vi "LTVUnicycleCtrl_New.vi"(8 "Max Velocity":dbl=9.0, 9 "dT":dbl=0.02, 10 "RELMS":T6=[[1.0], [2.0]], 11 "QELMS":T6=[[0.0625], [0.125], [0.2]]) -> (0 "Error":bool, 3 "LTV_UNICYCLE_CONTROLLER":T1={"States"=0, "Inputs"=0, "PoseError"={"TRANSLATION"={"X"=0.0, "Y"=0.0}, "ROTATION"={"VALUE"=0.0, "COS"=1.0, "SIN"=0.0}}, "PoseTolerance"={"TRANSLATION"={"X"=0.0, "Y"=0.0}, "ROTATION"={"VALUE"=0.0, "COS"=1.0, "SIN"=0.0}}, "Dt"=0.02, "Enabled"=FALSE, "LQR_K_Table"={"Table Xs"=[], "Table Ys"=[], "MinX"=0.0, "MaxX"=0.0, "ItemCount"=0, "Rows"=0, "Columns"=0}} {"PoseTolerance"."ROTATION"."SIN" format="%13.4f"; "PoseTolerance"."ROTATION"."COS" format="%13.4f"; "PoseTolerance"."ROTATION"."VALUE" format="%13.4f"; "PoseTolerance"."TRANSLATION"."Y" format="%14.3f"; "PoseTolerance"."TRANSLATION"."X" format="%14.3f"; "PoseError"."ROTATION"."SIN" format="%13.4f"; "PoseError"."ROTATION"."COS" format="%13.4f"; "PoseError"."ROTATION"."VALUE" format="%13.4f"; "PoseError"."TRANSLATION"."Y" format="%14.3f"; "PoseError"."TRANSLATION"."X" format="%14.3f"})   [LabVIEW 2019, in "Trajectory_Library.lvlib"]
doc: "The linear time-varying unicycle controller has a similar form to the LQR, but the model used to compute the controller gain is the nonlinear model linearized around the drivetrain's current state.\n\nConstructs a linear time-varying unicycle controller.\n\nInputs:\n - qelems -- The maximum desired error tolerance for each state. Matrix (3,1) Defaults (0.0625 m, 0.125 m, 0.2 rad)\n - relems -- The maximum desired control effort for each input. Matrix (2,1) Defaults (1 m/s, 2 rad/s)\n - dt -- Discretization timestep in seconds.\n - maxVelocity -- The maximum velocity in meters per second for the controller gain lookup table. (Option) The default is 9 m/s.\n\nOutputs:\n - LTV Unicycle Controller -- Created data structure.\n - Error -- If TRUE, an error occured."
uses:
  Trajectory_Library.lvlib
  <vilib>/Analysis/Matrix/Datatypes/RealMatrix.ctl
  TypeDef/LTV_UNICYCLE_CONTROLLER.ctl
  TypeDef/POSE2D.ctl
  TypeDef/TRANSLATION2D.ctl
  TypeDef/ROTATION2D.ctl
  TypeDef/FUNCTION_GENERATOR_MATRIX.ctl
  Enum/LTV_UNICYCLE_CONTROLLER_STATE_ENUM.ctl
  Rotation2d_CreateAngle.vi
  Translation2d_Create.vi
  MatrixHelper_CoerceSize.vi
  <vilib>/gmath/interp.llb/Search Ordered Table.vi
  <vilib>/Analysis/Matrix/NI_Matrix.lvlib
panel:
  # "<3,1>"
  # "<2, 1>"
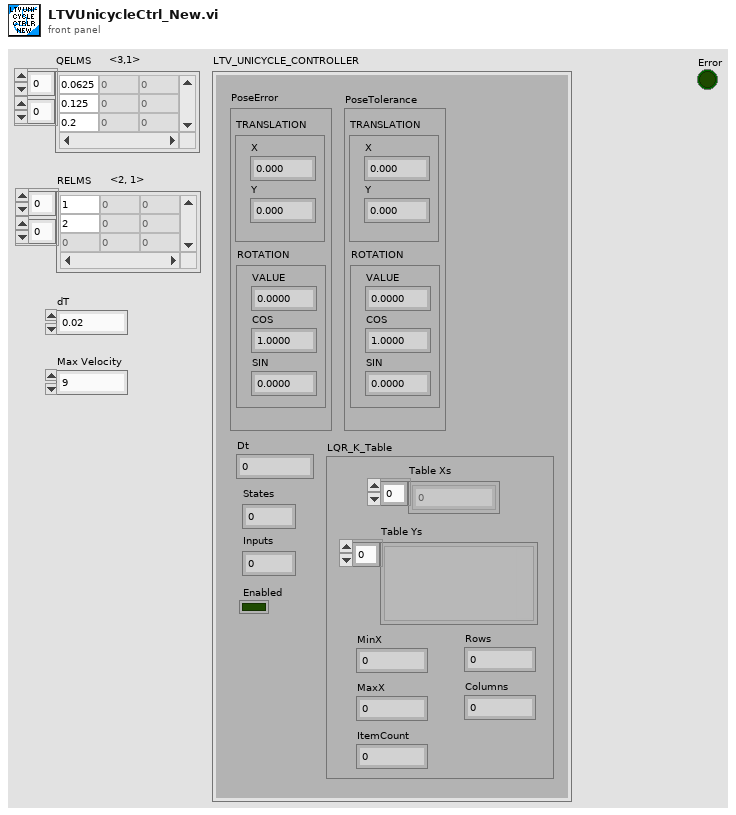
[diagram p1: front panel]
types:
  T1 = typedef "Trajectory_Library.lvlib/LTV_UNICYCLE_CONTROLLER.ctl" = cluster{"States":i32, "Inputs":i32, "PoseError":T2, "PoseTolerance":T2, "Dt":dbl, "Enabled":bool, "LQR_K_Table":T5}
  T2 = typedef "Trajectory_Library.lvlib/POSE2D.ctl" = cluster{"TRANSLATION":T3, "ROTATION":T4}
  T3 = typedef "Trajectory_Library.lvlib/TRANSLATION2D.ctl" = cluster{"X":dbl, "Y":dbl}
  T4 = typedef "Trajectory_Library.lvlib/ROTATION2D.ctl" = cluster{"VALUE":dbl, "COS":dbl, "SIN":dbl}
  T5 = typedef "Trajectory_Library.lvlib/FUNCTION_GENERATOR_MATRIX.ctl" = cluster{"Table Xs":dbl[], "Table Ys":variant[], "MinX":dbl, "MaxX":dbl, "ItemCount":i32, "Rows":i32, "Columns":i32}
  T6 = typedef "NI_Matrix.lvlib/RealMatrix.ctl" = dbl[][]
  T7 = typedef "Trajectory_Library.lvlib/LTV_UNICYCLE_CONTROLLER_STATE_ENUM.ctl" = enum16{"X", "Y", "HEADING"}
  T8 = typedef "Trajectory_Library.lvlib/LINEAR_QUADRATIC_REGULATOR.ctl" = cluster{"m_r":T6, "m_U":T6, "m_K":T6, "States":i32, "Inputs":i32}
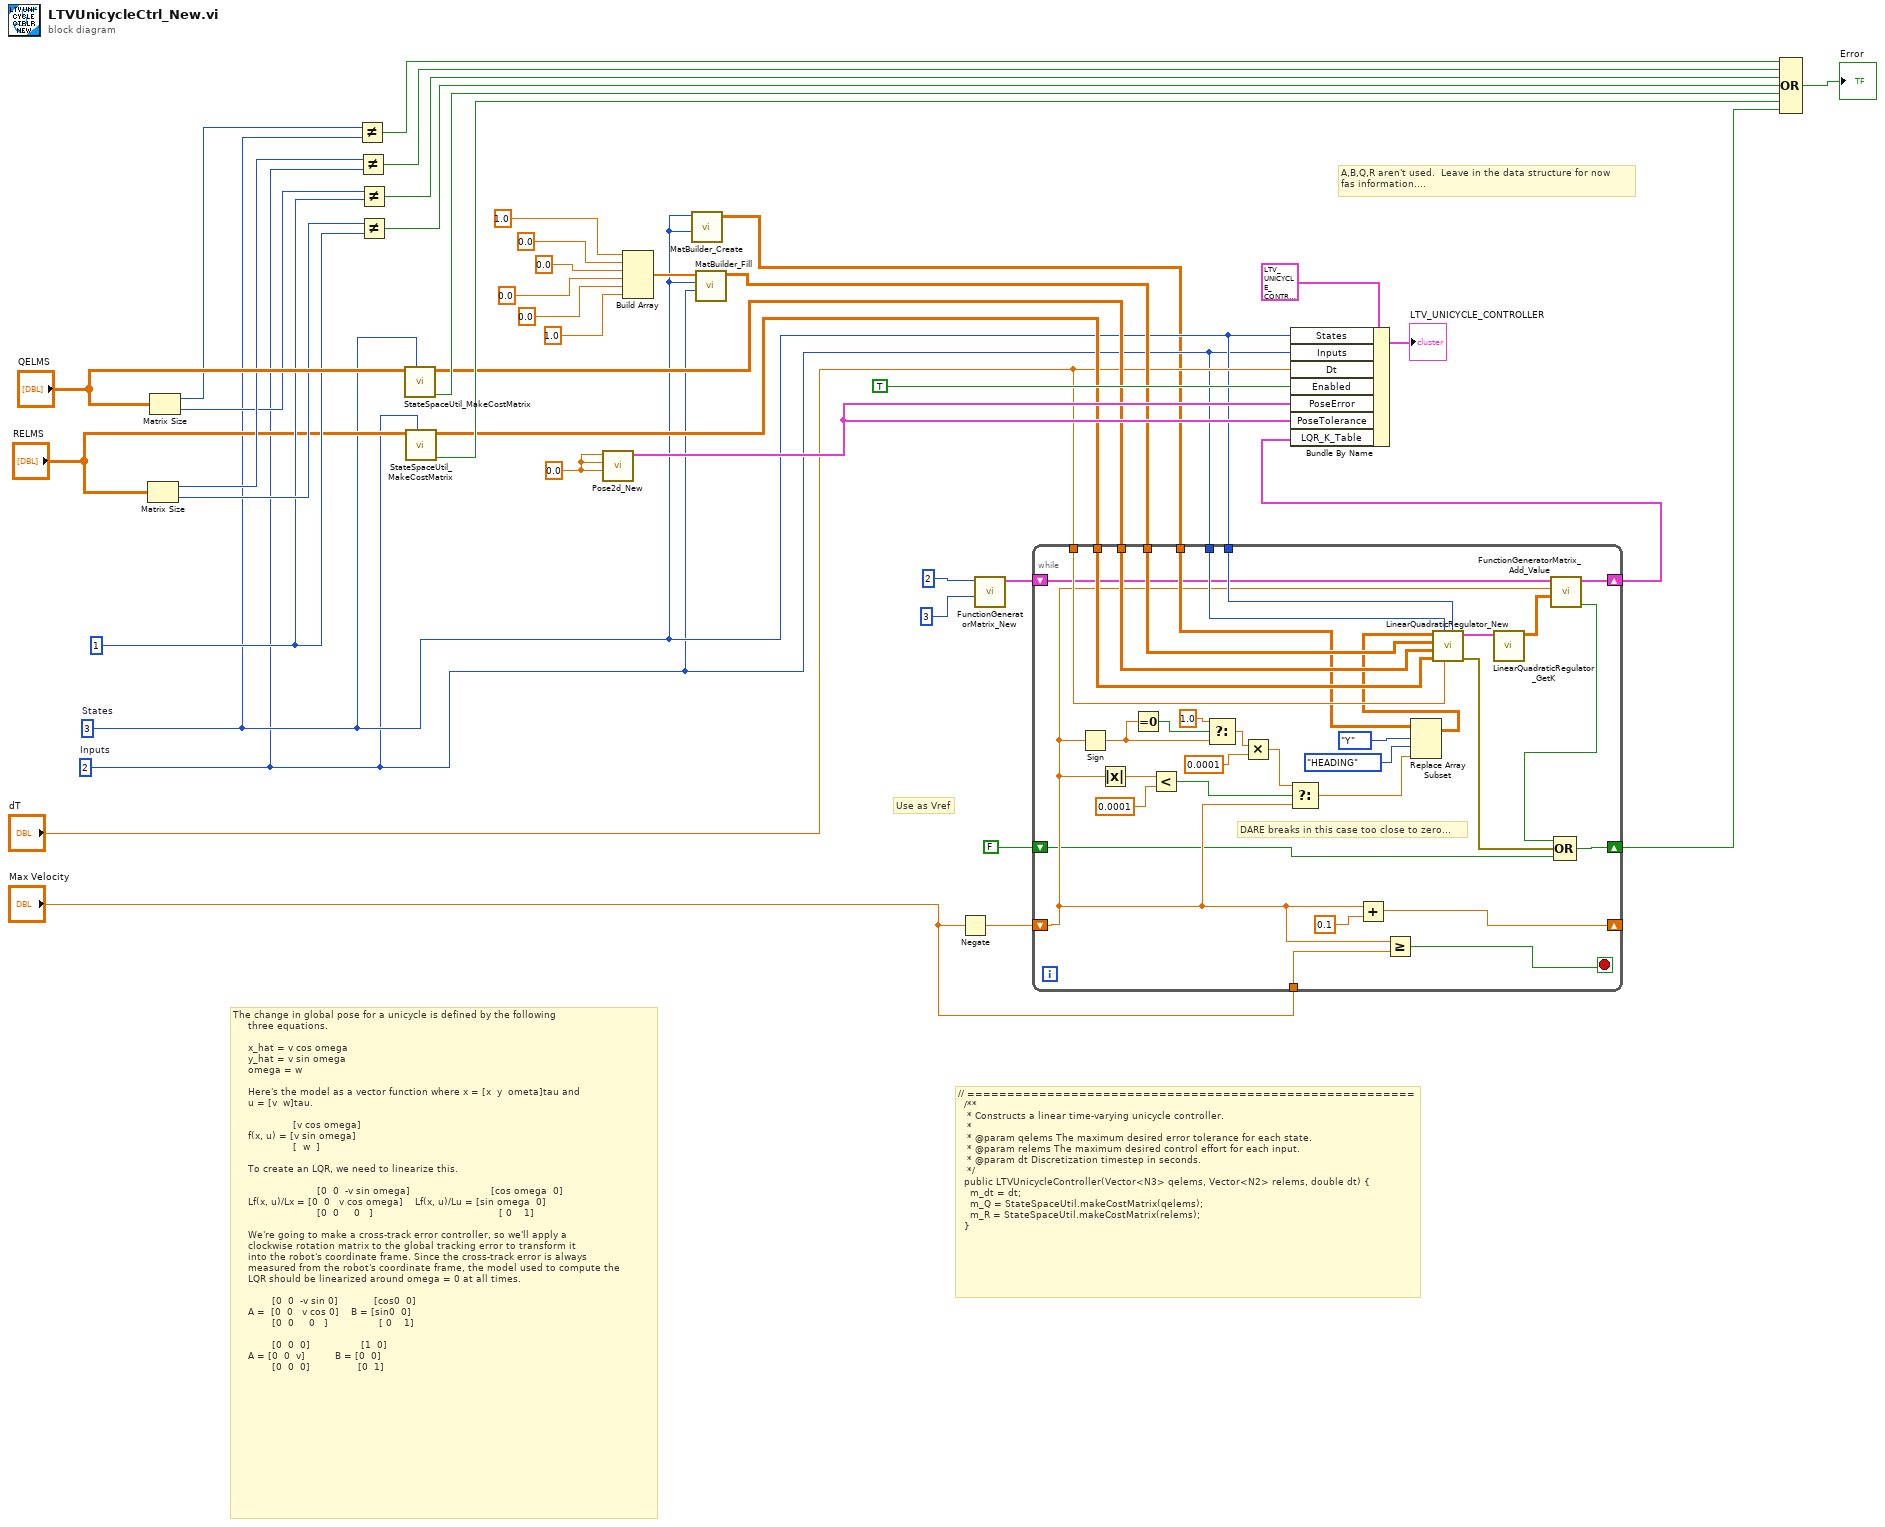
[diagram p0: block diagram]
diagram:
  w18 = 0.0 ("X")
  w8 = 2  # Inputs
  w9 = 3  # States
  w29 = 1 ("Columns")
  # "The change in global pose for a unicycle is defined by the following\n     three equations.\n    \n     x_hat = v cos omega\n     y_hat = v sin omega\n     omega = w\n    \n     Here's the model as a vector function where x = [x  y  ometa]tau and\n     u = [v  w]tau.\n    \n                    [v cos omega]\n     f(x, u) = [v sin omega]\n                    [  w  ]\n    \n     To create an LQR, we need to linearize this.\n    \n                            [0  0  -v sin omega]                           [cos omega  0]\n     Lf(x, u)/Lx = [0  0   v cos omega]    Lf(x, u)/Lu = [sin omega  0]\n                            [0  0     0   ]                                          [ 0    1]\n    \n     We're going to make a cross-track error controller, so we'll apply a\n     clockwise rotation matrix to the global tracking error to transform it\n     into the robot's coordinate frame. Since the cross-track error is always\n     measured from the robot's coordinate frame, the model used to compute the\n     LQR should be linearized around omega = 0 at all times.\n    \n             [0  0  -v sin 0]            [cos0  0]\n     A =  [0  0   v cos 0]    B = [sin0  0]\n             [0  0     0   ]                 [ 0    1]\n    \n             [0  0  0]                 [1  0]\n     A = [0  0  v]          B = [0  0]\n             [0  0  0]                [0  1]"
  # "A,B,Q,R aren't used.  Leave in the data structure for now\nfas information...."
  # "Use as Vref"
  # "// ========================================================\n  /**\n   * Constructs a linear time-varying unicycle controller.\n   *\n   * @param qelems The maximum desired error tolerance for each state.\n   * @param relems The maximum desired control effort for each input.\n   * @param dt Discretization timestep in seconds.\n   */\n  public LTVUnicycleController(Vector<N3> qelems, Vector<N2> relems, double dt) {\n    m_dt = dt;\n    m_Q = StateSpaceUtil.makeCostMatrix(qelems);\n    m_R = StateSpaceUtil.makeCostMatrix(relems);\n  }"
  n1 = Matrix Size(0:"RELMS") -> (1:w32:i32, 2:w30:i32)
  n2 = Matrix Size(0:"QELMS") -> (1:w33:i32, 2:w31:i32)
  n3 = Not Equal?(x=w33, y=w9) -> (x != y?=w41:bool)
  n4 = Not Equal?(x=w32, y=w8) -> (x != y?=w39:bool)
  n5 = Not Equal?(x=w31, y=w29) -> (x != y?=w38:bool)
  n6 = Not Equal?(x=w30, y=w29) -> (x != y?=w37:bool)
  n7 = call "StateSpaceUtil_MakeCostMatrix.vi"("Elements"=w9, "Costs"="QELMS") -> ("Sze Coerced"=w28:bool, "Costs Matrix"=w12:T6)  [unwired: 8 in]
  n8 = call "StateSpaceUtil_MakeCostMatrix.vi"("Elements"=w8, "Costs"="RELMS") -> ("Sze Coerced"=w27:bool, "Costs Matrix"=w11:T6)  [unwired: 8 in]
  n9 = call "Pose2d_New.vi"("Heading"=w18, "Y"=w18, "X"=w18) -> ("out POSe"=w17:T2)  [unwired: 8 in]
  n10 = Build Array(1.0 ("element"), 0.0 ("element"), 0.0 ("element"), 0.0 ("element"), 0.0 ("element"), 1.0 ("element")) -> (w26:dbl[])
  n11 = call "MatBuilder_Create.vi"("Columns"=w9, "Rows"=w9) -> ("output matrix"=w7:T6)  [unwired: 9 in]
  n12 = call "MatBuilder_Fill.vi"("Columns"=w8, "Rows"=w9, "Value List"=w26) -> ("output matrix"=w13:T6)  [unwired: 8 in]
  n13 = Negate(x="Max Velocity") -> (-x=w15:dbl)
  n14 = call "FunctionGeneratorMatrix_New.vi"("Columns"=3, "Rows"=2) -> ("FUNCTION_GENERATOR_MATRIX"=w14:T5)  [unwired: 9 in]
  n15 = while {
    shift-right: [w71] -> _
    shift-left: w15 -> [w52]
    tunnel: "Max Velocity" -> [w73]
    tunnel: w13 -> [w70]
    tunnel: w12 -> [w69]
    tunnel: w11 -> [w68]
    tunnel: "dT" -> [w67]
    tunnel: w9 -> [w66]
    tunnel: w8 -> [w65]
    tunnel: w7 -> [w56]
    shift-right: [w53] -> w6
    shift-left: w14 -> [w50]
    shift-right: [w48] -> w2
    shift-left: FALSE -> [w49]
    stop <- w72 stop-if-true
    # "DARE breaks in this case too close to zero..."
    n16 = Sign(1:w52) -> (0:w42:dbl)
    n17 = Absolute Value(x=w52) -> (abs(x)=w64:dbl)
    n18 = Equal To 0?(x=w42) -> (x = 0?=w43:bool)
    n19 = Less?(x=w64, y=0.0001) -> (x < y?=w62:bool)
    n20 = Select(t=1.0, s=w43, f=w42) -> (s? t:f=w45:dbl)
    n21 = Multiply(x=w45, y=0.0001 ("t")) -> (x*y=w61:dbl)
    n22 = Select(t=w61, s=w62, f=w52) -> (s? t:f=w57:dbl)
    n23 = Add(x=w52, y=0.1) -> (x+y=w71:dbl)
    n24 = Greater Or Equal?(x=w52, y=w73) -> (x >= y?=w72:bool)
    n25 = Replace Array Subset(array=w56, new element=w57, index (row)=LTV_UNICYCLE_CONTROLLER_STATE_ENUM."Y" ("LTV_UNICYCLE_CONTROLLER_STATE"), index (col)=LTV_UNICYCLE_CONTROLLER_STATE_ENUM."HEADING" ("LTV_UNICYCLE_CONTROLLER_STATE")) -> (w55:T6)
    n26 = call "LinearQuadraticRegulator_New.vi"("States"=w66, "dt_Seconds"=w67, "Inputs"=w65, "R"=w68, "Q"=w69, "B"=w70, "A"=w55) -> ("Error"=w47:errorcluster, "LinearQuadraticRegulator"=w54:T8)  [unwired: 3 in]
    n27 = call "LinearQuadraticRegulator_GetK.vi"("in LinearQuadraticRegulator"=w54) -> ("K"=w51:T6)  [unwired: 10 in]
    n28 = call "FunctionGeneratorMatrix_Add_Value.vi"("Y Value"=w51, "X Value"=w52, "in FUNC_GEN_MATRIX"=w50) -> ("Error"=w46:bool, "out FUNC_GEN_MATRIX"=w53:T5)  [unwired: 7 in]
    n29 = Compound Arithmetic op=OR(w46, w47, w49) -> (w48:bool)
  }
  n30 = Bundle By Name(cluster=T1 {"States"=0, "Inputs"=0, "PoseError"={"TRANSLATION"={"X"=0.0, "Y"=0.0}, "ROTATION"={"VALUE"=0.0, "COS"=1.0, "SIN"=0.0}}, "PoseTolerance"={"TRANSLATION"={"X"=0.0, "Y"=0.0}, "ROTATION"={"VALUE"=0.0, "COS"=1.0, "SIN"=0.0}}, "Dt"=0.02, "Enabled"=FALSE, "LQR_K_Table"={"Table Xs"=[], "Table Ys"=[], "MinX"=0.0, "MaxX"=0.0, "ItemCount"=0, "Rows"=0, "Columns"=0}} ("LTV_UNICYCLE_CONTROLLER"), "States"=w9, "Inputs"=w8, "Dt"="dT", "Enabled"=TRUE, "PoseError"=w17, "PoseTolerance"=w17, "LQR_K_Table"=w6) -> (→"LTV_UNICYCLE_CONTROLLER":T1)
  n31 = Compound Arithmetic op=OR(w41, w39, w38, w37, w28, w27, w2) -> (→"Error":bool)
